vi "Set Operation Parameters.vi"(4 "Run Parameters":T2={"Run Mode"=0, "Volume Value"=1.0, "Volume Unit"=1, "Infuse Flowrate Value"=1.0, "Infuse Flowrate Unit"=1, "Withdraw Flowrate Value"=1.0, "Withdraw Flowrate Unit"=1, "Interval Time 1 Value"=100.0, "Interval Time 1 Unit"=2, "Interval Time 2 Value"=1.0, "Interval Time 2 Unit"=2, "Drive Force"=100, "Drive Force Unit"=0, "Dispensing Times"=1, "Run Cycles"=1} caption="运行参数" {"Drive Force Unit" items=["%"]; "Run Cycles" step=1; "Dispensing Times" min=1 max=9999 step=1; "Drive Force" max=100 step=1; "Interval Time 2 Unit" items=["h", "min", "s"]; "Interval Time 1 Unit" items=["h", "min", "s"]; "Interval Time 2 Value" min=0.001; "Interval Time 1 Value" min=0.001; "Run Mode" items=["灌注模式", "抽取模式", "灌注/抽取模式", "抽取/灌注模式"]; "Withdraw Flowrate Unit" items=["L/min", "mL/min", "uL/min", "nL/min"]; "Withdraw Flowrate Value" min=0.001; "Infuse Flowrate Unit" items=["L/min", "mL/min", "uL/min", "nL/min"]; "Infuse Flowrate Value" min=0.001; "Volume Unit" items=["L", "mL", "uL", "nL"]; "Volume Value" min=0.001}, 6 "Syringe Configuration":T1={"Syringe Speicification"=100.0, "Volume Unit"=2, "Syringe Stroke"=57.1513, "Syringe Length Unit"=0} caption="注射器配置" {"Syringe Length Unit" items=["mm"]; "Syringe Stroke" min=0.001; "Volume Unit" items=["mL"=1, "uL"=2]; "Syringe Speicification" min=0.001}, 8 "Error in":errorcluster caption="错误输入", 10 "Channel":dbl=1.0 caption="设备通道", 11 "Modbus master in":refnum<class "Modbus Master.lvclass"> caption="Modbus实例输入") -> (0 "Error out":errorcluster caption="错误输出", 3 "Modbus instance out":refnum<class "Modbus API.lvclass"> caption="Modbus实例输出")   [LabVIEW 2023, in "Longer Pump dLSP501 Series.lvlib"]
uses:
  <instrlib>/Longer Pump dLSP501 Modbus RTU Series/Longer Pump dLSP501 Series.lvlib
  <vilib>/NI/Modbus Library/API/Modbus API.lvclass
  <vilib>/NI/Modbus Library/API/Master/Modbus Master.lvclass
  C:/Program Files/National Instruments/LabVIEW 2023/vi.lib/NI/Modbus Library/API/Modbus API.lvclass
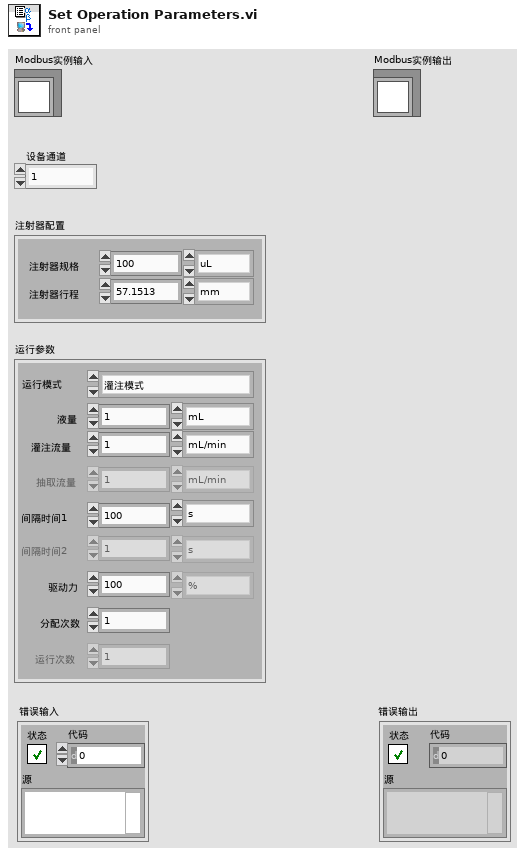
[diagram p1: front panel]
types:
  T1 = cluster{"Syringe Speicification":dbl, "Volume Unit":u16, "Syringe Stroke":dbl, "Syringe Length Unit":u16}
  T2 = cluster{"Run Mode":u16, "Volume Value":dbl, "Volume Unit":u16, "Infuse Flowrate Value":dbl, "Infuse Flowrate Unit":u16, "Withdraw Flowrate Value":dbl, "Withdraw Flowrate Unit":u16, "Interval Time 1 Value":dbl, "Interval Time 1 Unit":u16, "Interval Time 2 Value":dbl, "Interval Time 2 Unit":u16, "Drive Force":u16, "Drive Force Unit":u16, "Dispensing Times":u16, "Run Cycles":u16}
  T3 = enum8{"Enabled", "Disabled", "Disabled and Grayed Out"}
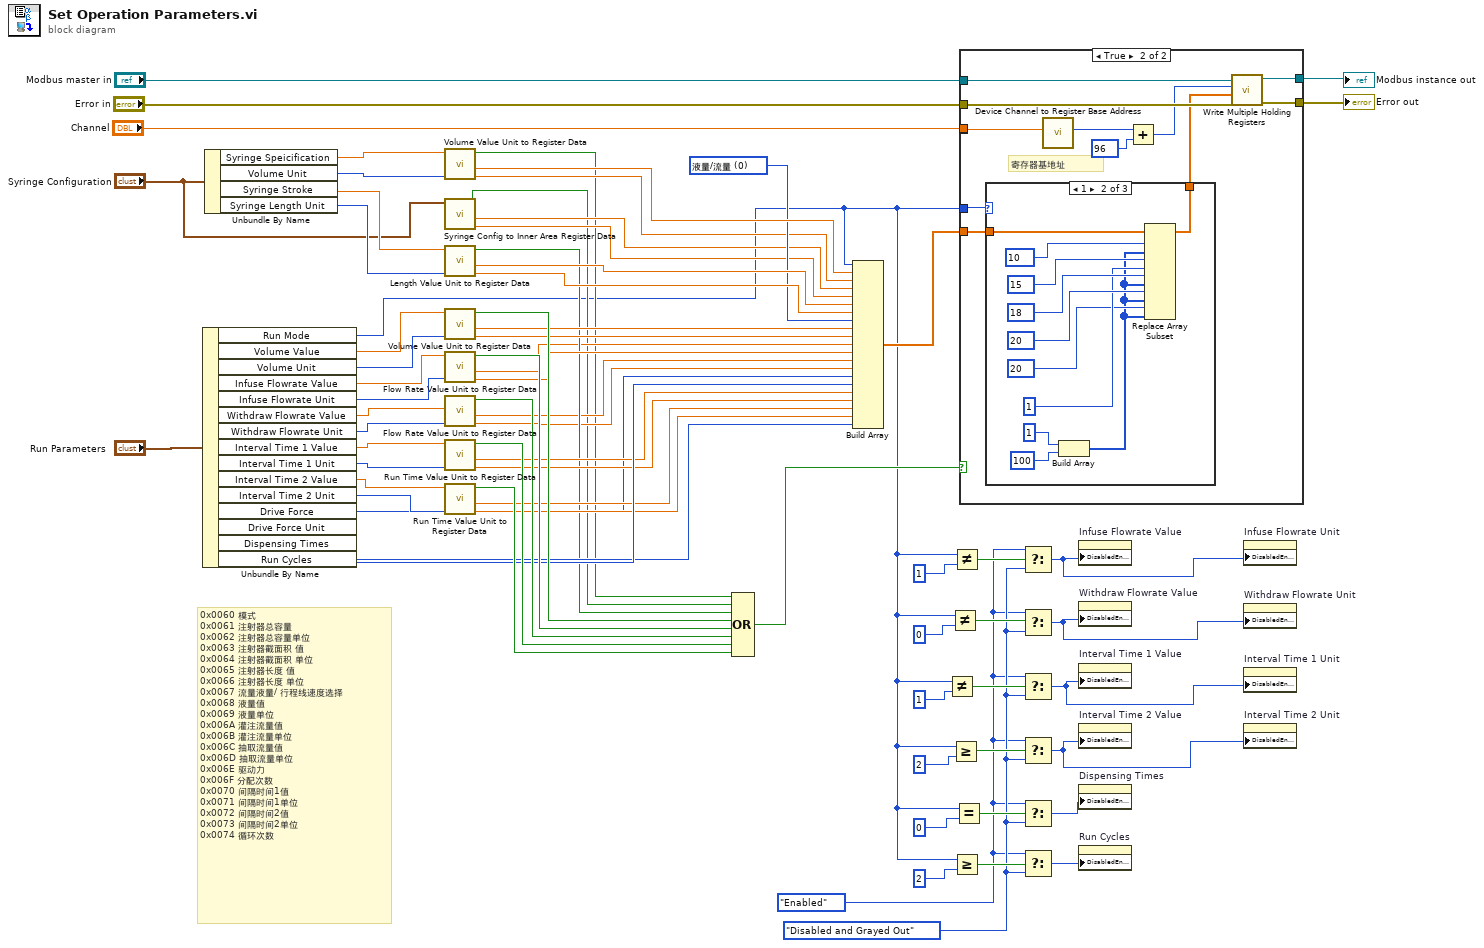
[diagram p0: block diagram]
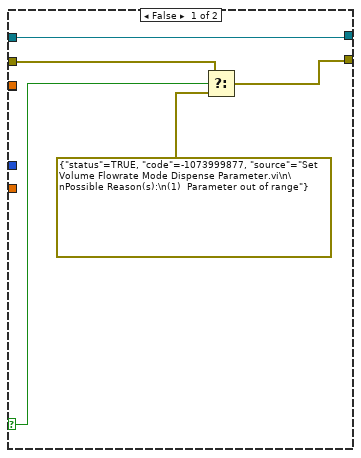
[diagram p2: hidden frame]
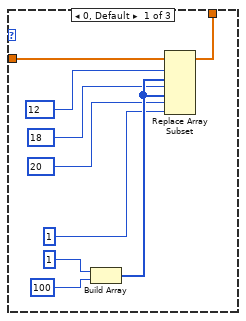
[diagram p3: hidden frame]
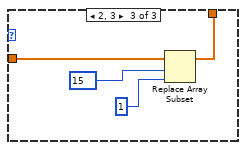
[diagram p4: hidden frame]
diagram:
  w5 = T3."Disabled and Grayed Out" ("禁用")
  w4 = T3."Enabled" ("禁用")
  w38 = u16 0 items=["液量/流量", "速度"]
  # "0x0060\t模式\n0x0061\t注射器总容量\n0x0062\t注射器总容量单位\n0x0063\t注射器截面积 值\n0x0064\t注射器截面积 单位\n0x0065\t注射器长度 值\n0x0066\t注射器长度 单位\n0x0067\t流量液量/ 行程线速度选择\n0x0068\t液量值\n0x0069\t液量单位\n0x006A\t灌注流量值\n0x006B\t灌注流量单位\n0x006C\t抽取流量值\n0x006D\t抽取流量单位\n0x006E\t驱动力\n0x006F\t分配次数\n0x0070\t间隔时间1值\n0x0071\t间隔时间1单位\n0x0072\t间隔时间2值\n0x0073\t间隔时间2单位\n0x0074\t循环次数"
  n1 = Unbundle By Name("Run Parameters") -> ("Run Mode"=w1:u16, "Volume Value"=w69:dbl, "Volume Unit"=w68:u16, "Infuse Flowrate Value"=w67:dbl, "Infuse Flowrate Unit"=w66:u16, "Withdraw Flowrate Value"=w65:dbl, "Withdraw Flowrate Unit"=w64:u16, "Interval Time 1 Value"=w63:dbl, "Interval Time 1 Unit"=w62:u16, "Interval Time 2 Value"=w61:dbl, "Interval Time 2 Unit"=w60:u16, "Drive Force"=w28:u16, "Dispensing Times"=w50:u16, "Run Cycles"=w45:u16)  [unwired: 1 out]
  n2 = Unbundle By Name("Syringe Configuration") -> ("Syringe Speicification"=w43:dbl, "Volume Unit"=w42:u16, "Syringe Stroke"=w35:dbl, "Syringe Length Unit"=w34:u16)
  n3 = call <instrlib>:"Volume Value Unit to Register Data.vi"("Volume Value"=w43, "Volume Unit"=w42) -> ("Valid Result"=w27:bool, "Value Reg Data"=w41:dbl, "Unit Reg Data"=w36:dbl)  [unwired: 6 in]
  n4 = call <instrlib>:"Syringe Config to Inner Area Register Data.vi"("Syringe Configuration"="Syringe Configuration") -> ("Valid Result"=w26:bool, "Value Reg Data"=w33:dbl, "Unit Reg Data"=w32:dbl)  [unwired: 7 in]
  n5 = call <instrlib>:"Length Value Unit to Register Data.vi"("Length Value"=w35, "Length Unit"=w34) -> ("Valid Result"=w37:bool, "Value Reg Data"=w40:dbl, "Unit Reg Data"=w39:dbl)  [unwired: 6 in]
  n6 = call <instrlib>:"Volume Value Unit to Register Data.vi"("Volume Value"=w69, "Volume Unit"=w68) -> ("Valid Result"=w58:bool, "Value Reg Data"=w53:dbl, "Unit Reg Data"=w52:dbl)  [unwired: 6 in]
  n7 = call <instrlib>:"Flow Rate Value Unit to Register Data.vi"("Flow Rate Value"=w67, "Flow Rate Unit"=w66) -> ("Valid Result"=w57:bool, "Value Reg Data"=w31:dbl, "Unit Reg Data"=w51:dbl)  [unwired: 6 in]
  n8 = call <instrlib>:"Flow Rate Value Unit to Register Data.vi"("Flow Rate Value"=w65, "Flow Rate Unit"=w64) -> ("Valid Result"=w56:bool, "Value Reg Data"=w29:dbl, "Unit Reg Data"=w30:dbl)  [unwired: 6 in]
  n9 = call <instrlib>:"Run Time Value Unit to Register Data.vi"("Run Time Value"=w63, "Run Time Unit"=w62) -> ("Valid Result"=w55:bool, "Value Reg Data"=w49:dbl, "Unit Reg Data"=w48:dbl)  [unwired: 6 in]
  n10 = call <instrlib>:"Run Time Value Unit to Register Data.vi"("Run Time Value"=w61, "Run Time Unit"=w60) -> ("Valid Result"=w54:bool, "Value Reg Data"=w47:dbl, "Unit Reg Data"=w46:dbl)  [unwired: 6 in]
  n11 = Compound Arithmetic op=OR ("复合运算")(w27, w26, w37, w58, w57, w56, w55, w54) -> (w59:bool)
  n12 = Build Array(w1, w41, w36, w33, w32, w40, w39, w38, w53, w52, w31, w51, w29, w30, w28, w50, w49, w48, w47, w46, w45) -> (w44:dbl[])
  n13 = Not Equal?(x=w1, y=u16 1) -> (x != y?=w17:bool)
  n14 = Not Equal?(x=w1, y=u16 0) -> (x != y?=w14:bool)
  n15 = Greater Or Equal?(x=w1, y=u16 2) -> (x >= y?=w22:bool)
  n16 = Not Equal?(x=w1, y=u16 1) -> (x != y?=w15:bool)
  n17 = Greater Or Equal?(x=w1, y=u16 2) -> (x >= y?=w23:bool)
  n18 = Equal?(x=w1, y=u16 0) -> (x = y?=w12:bool)
  n19 = case shown="True" w59 {
    selector: w59 -> [w76 _]
    tunnel: "Error in" -> [w75 w88]
    tunnel: w44 -> [_ w84]
    tunnel: "Modbus master in" -> [w77 w87]
    tunnel: [w74 w86] -> w2
    tunnel: [w77 w85] -> w70
    tunnel: w1 -> [_ w78]
    tunnel: [_ w82] -> _
    tunnel: "Channel" -> [_ w82]
    frame False {
      n20 = Select(t=w75, s=w76, f=errorcluster {"status"=TRUE, "code"=-1073999877, "source"="Set Volume Flowrate Mode Dispense Parameter.vi\n\nPossible Reason(s):\n(1)  Parameter out of range"} ("t")) -> (s? t:f=w74:errorcluster)
    }
    frame True {
      # "寄存器基地址"
      n21 = case shown="1" w78 {
        tunnel: w84 -> [w94 w108 w111]
        tunnel: [w93 w107 w110] -> w83
        frame 0, Default {
          n22 = Build Array(1, 100) -> (w92:i32[])
          n23 = Replace Array Subset(array=w94, new element #1=w92, index #1=u16 12 ("starting address"), new element #2=w92, index #2=u16 18 ("starting address"), new element #3=1, index #3=u16 20 ("starting address")) -> (w93:dbl[])
        }
        frame 1 {
          n24 = Build Array(1, 100) -> (w98:i32[])
          n25 = Replace Array Subset(array=w108, new element #1=w98, index #1=u16 10 ("starting address"), new element #2=1, index #2=u16 15 ("starting address"), new element #3=w98, index #3=u16 18 ("starting address"), new element #4=w98, index #4=u16 20 ("starting address"), new element #5=w98, index #5=u16 20 ("starting address")) -> (w107:dbl[])
        }
        frame 2, 3 {
          n26 = Replace Array Subset(array=w111, new element=1, index=u16 15 ("starting address")) -> (w110:dbl[])
        }
      }
      n27 = call <instrlib>:"Device Channel to Register Base Address.vi"("Channel"=w82) -> ("Register Base Address"=w80:u16)  [unwired: 10 in]
      n28 = Add(x=w80, y=u16 96 ("address")) -> (x+y=w81:u16)
      n29 = call-dynamic "Write Multiple Holding Registers.vi"("error in"=w88, "registers to write"=w83, "starting address"=w81, "Modbus master in"=w87) -> ("error out"=w86:errorcluster, "Modbus master out"=w85:refnum<class "Modbus Master.lvclass">)  [unwired: 6 in]
    }
  }
  "Modbus instance out" <- w70
  "Error out" <- w2
  n30 = Select(t=w4, s=w15, f=w5) -> (s? t:f=w18:T3)
  n31 = Select(t=w4, s=w14, f=w5) -> (s? t:f=w19:T3)
  n32 = Select(t=w4, s=w17, f=w5) -> (s? t:f=w20:T3)
  n33 = Select(t=w4, s=w22, f=w5) -> (s? t:f=w21:T3)
  n34 = Select(t=w4, s=w12, f=w5) -> (s? t:f=w13:T3)
  n35 = Select(t=w4, s=w23, f=w5) -> (s? t:f=w16:T3)
  n36 = property on="Infuse Flowrate Value" class="DigNum (strict)"("DisabledEnum"=w18) -> ()  [unwired: 2 in, 2 out]
  n37 = property on="Withdraw Flowrate Value" class="DigNum (strict)"("DisabledEnum"=w19) -> ()  [unwired: 2 in, 2 out]
  n38 = property on="Interval Time 1 Value" class="DigNum (strict)"("DisabledEnum"=w20) -> ()  [unwired: 2 in, 2 out]
  n39 = property on="Interval Time 2 Value" class="DigNum (strict)"("DisabledEnum"=w21) -> ()  [unwired: 2 in, 2 out]
  n40 = property on="Dispensing Times" class="DigNum (strict)"("DisabledEnum"=w13) -> ()  [unwired: 2 in, 2 out]
  n41 = property on="Run Cycles" class="DigNum (strict)"("DisabledEnum"=w16) -> ()  [unwired: 2 in, 2 out]
  n42 = property on="Infuse Flowrate Unit" class="Ring (strict)"("DisabledEnum"=w18) -> ()  [unwired: 2 in, 2 out]
  n43 = property on="Withdraw Flowrate Unit" class="Ring (strict)"("DisabledEnum"=w19) -> ()  [unwired: 2 in, 2 out]
  n44 = property on="Interval Time 1 Unit" class="Ring (strict)"("DisabledEnum"=w20) -> ()  [unwired: 2 in, 2 out]
  n45 = property on="Interval Time 2 Unit" class="Ring (strict)"("DisabledEnum"=w21) -> ()  [unwired: 2 in, 2 out]
